vi "Actor Destroy.vi"(11 "Self Actor in":refnum<class "Self Actor.lvclass">) -> (3 "Self Actor out":refnum<class "Self Actor.lvclass">)   [LabVIEW 2021, in "jettl.lvlib" / "Self Actor.lvclass"]
uses:
  Self Actor.lvclass
  C:/git/jettl/src_error_internal/LVCAM/LVCAM/Actor/Actor.lvclass
  Destroying Self Actor State/Destroying Self Actor State.lvclass
  C:/git/jettl/src_error_internal/LVCAM/LVCAM/Self Actor State/Self Actor State.lvclass
  Self Actor.lvclass/Self Actor.ctl
  Self Actor State/Self Actor State.lvclass
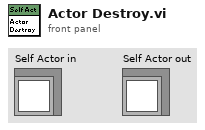
[diagram p1: front panel]
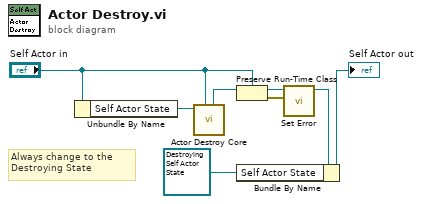
[diagram p0: block diagram]
diagram:
  # "Always change to the Destroying State"
  n1 = Unbundle By Name("Self Actor in") -> ("Self Actor State"=w7:refnum<class "Self Actor State.lvclass">)
  n2 = call-dynamic "Actor Destroy Core.vi"("Actor in"="Self Actor in", "Self Actor State in"=w7) -> ("Actor out"=w5:refnum<class "Actor.lvclass">)  [unwired: 9 in]
  n3 = Preserve Run-Time Class(object in=w5, 2:"Self Actor in") -> (object out=w3:refnum<class "Self Actor.lvclass">, error out=w1:errorcluster)  [unwired: 1 in]
  n4 = call-dynamic "Set Error.vi"("Error"=w1, "Self Actor in"=w3) -> ("Self Actor out"=w2:refnum<class "Self Actor.lvclass">)  [unwired: 9 in]
  n5 = Bundle By Name(cluster=w2, "Self Actor State"=refnum<class "Destroying Self Actor State.lvclass"> refnum ("LVCAM.lvlib:Destroying Self Actor State.lvclass")) -> (→"Self Actor out":refnum<class "Self Actor.lvclass">)
